vi "PPMSDR_write_single_file_post.vi"() -> ()   [LabVIEW 2013]
uses:
  <vilib>/lvdsc/historical/Open Trace (Numeric).vi
  <vilib>/lvdsc/historical/Write Trace (Numeric).vi
  <vilib>/lvdsc/NI_DSC.lvlib
panel:
  in  "file path (dialog if empty)":path=path "\\\\PPMS\\Data/logppmsdata_20160829.dat"
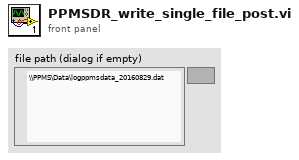
[diagram p1: front panel]
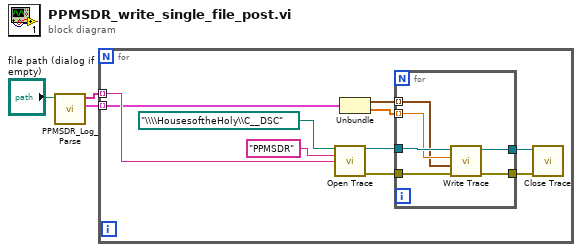
[diagram p0: block diagram]
diagram:
  n1 = call "PPMSDR_Log_Parse.vi"("file path (dialog if empty)"="file path (dialog if empty)") -> ("Array 2"=w2:cluster{timestamp[], dbl[]}[], "Array"=w3:string[])  [unwired: 9 in]
  n2 = for {
    tunnel: w3 -> [w7] mode=indexing
    tunnel: w2 -> [w6] mode=indexing
    n3 = call-poly <vilib>:"Open Trace.vi"("database URL"=path "\\\\HousesoftheHoly\\C__DSC", "process name"="PPMSDR", "trace name"=w7) -> ("trace reference"=w9:refnum<k1>, "error out"=w8:errorcluster)  [unwired: 10 in, 1 out]
    n4 = Unbundle(w6) -> (w5:timestamp[], w4:dbl[])
    n5 = for {
      tunnel: [w19] -> w11
      tunnel: [w18] -> w10
      tunnel: w9 -> [w17]
      tunnel: w8 -> [w16]
      tunnel: w5 -> [w14] mode=indexing
      tunnel: w4 -> [w15] mode=indexing
      n6 = call-poly <vilib>:"Write Trace.vi"("error in (no error)"=w16, "timestamp (now)"=w14, "value"=w15, "trace ref"=w17) -> ("error out"=w19:errorcluster, "trace ref out"=w18:refnum<k1>)  [unwired: 6 in]
    }
    n7 = call <vilib>:"Close Trace.vi"("error in (no error)"=w11, "trace reference"=w10) -> ()  [unwired: 9 in, 1 out]
  }
